vi "TPNT_GetTypes.vi"(11 "Objects":T1[](array[typedef])) -> (2 "types":string)   [LabVIEW 2016]
uses:
  TPNT_Refnum.ctl
  TPNT_CoreFunction.ctl
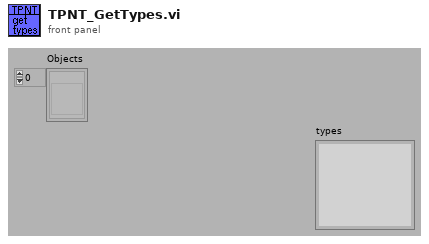
[diagram p1: front panel]
types:
  T1 = typedef "TPNT_Refnum.ctl" = refnum<vi>
  T2 = typedef "TPNT_CoreFunction.ctl" = enum16{"Reset", "Register", "Get Data", "Set Data", "Unregister", "Test", "Get Objects"}
  T3 = typedef "TPNT_DeviceTPs.ctl" = cluster{"device":string, "devupdate":dbl, "next_update":u32, "devinterface":string, "TPs":T4[], "Alarms":bool, "monitor":bool, "log sep":string}
  T4 = typedef "TPNT_TP.ctl" = cluster{"name":string, "type":string, "algor":string[], "update_rate":sgl, "Limits":T5, "Samples":T6, "next_update":u32, "Status":string, "monitor":bool, "error":bool, "Log":T7, "permissions":string, "ID":string}
  T5 = typedef "TPNT_Limits.ctl" = cluster{"Alarm Type":string, "Lower ":dbl, "Upper":dbl, "Nominal":dbl, "outrange":bool, "Check":bool, "latch":bool, "level":string}
  T6 = typedef "TPNT_Samples.ctl" = cluster{"samples":i32, "counter":i32, "Values":dbl[], "Current Value":string, "filter":string, "precision":u8}
  T7 = typedef "TPNT_Log.ctl" = cluster{"log":bool, "file":path, "type":string, "format":string, "updaterate":dbl, "nex_update":u32, "mode":string}
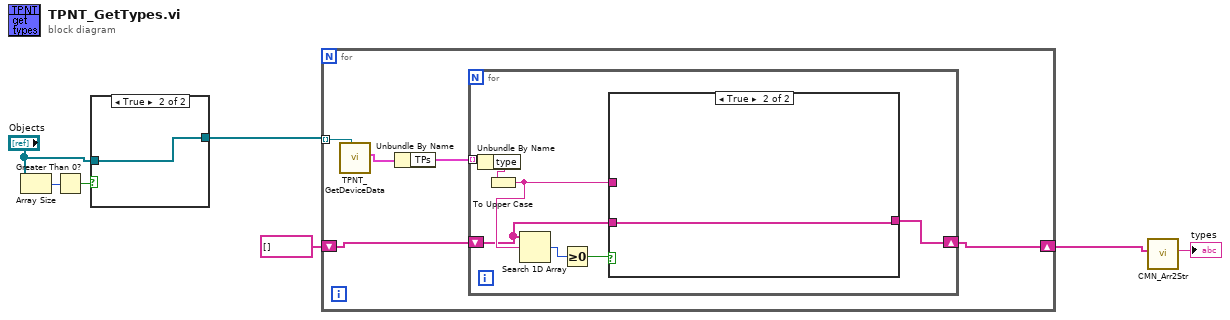
[diagram p0: block diagram]
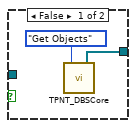
[diagram p2: hidden frame]
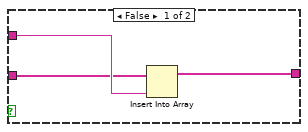
[diagram p3: hidden frame]
diagram:
  n1 = Array Size(array="Objects") -> (size(s)=w6:i32)
  n2 = Greater Than 0?(x=w6) -> (x > 0?=w5:bool)
  n3 = case shown="True" w5 {
    tunnel: [w8 w10] -> w7
    tunnel: "Objects" -> [_ w10]
    frame False {
      n4 = call "TPNT_DBSCore.vi"("Function (Get Data)"=TPNT_CoreFunction."Get Objects") -> ("Objects"=w8:T1[])  [unwired: 4 in, 14 out]
    }
    frame True {
    }
  }
  n5 = for {
    tunnel: w7 -> [w15] mode=indexing
    shift-right: [w12] -> w2
    shift-left: string[] [] -> [w11]
    n6 = call "TPNT_GetDeviceData.vi"("Object Refnum In"=w15) -> ("Object Data Out"=w14:T3)  [unwired: 1 in, 9 out]
    n7 = Unbundle By Name(w14) -> ("TPs"=w13:T4[])
    n8 = for {
      tunnel: w13 -> [w22] mode=indexing
      shift-right: [w20] -> w12
      shift-left: w11 -> [w16]
      n9 = Unbundle By Name(w22) -> ("type"=w21:string)
      n10 = To Upper Case(1:w21) -> (0:w19:string)
      n11 = Search 1D Array(1D array=w16, element=w19) -> (index of element=w18:i32)  [unwired: 1 in]
      n12 = Greater Or Equal To 0?(x=w18) -> (x >= 0?=w17:bool)
      n13 = case shown="True" w17 {
        tunnel: w19 -> [w25 _]
        tunnel: [w24 w26] -> w20
        tunnel: w16 -> [w23 w26]
        frame False {
          n14 = Insert Into Array(array=w23, new element=w25) -> (w24:string[])  [unwired: 1 in]
        }
        frame True {
        }
      }
    }
  }
  n15 = call "CMN_Arr2Str.vi"("Array in"=w2) -> ("string out"=→"types":string)  [unwired: 10 out]
